vi "ROI to Default ROI Name.vi"(8 "Error In":errorcluster, 11 "ROI":T1) -> (0 "Error Out":errorcluster, 3 "ROI Type String":string)   [LabVIEW 2021, in "Image.lvlib"]
uses:
  Image.lvlib
panel:
  in  "Type":u32(ring)=1 items=["No Selection", "Point", "Line", "Rectangle", "Oval", "Polygon", "Free", "Annulus", "Unused2", "Unused3", "Broken Line", "Free Hand Line", "Rotated Rectangle"]
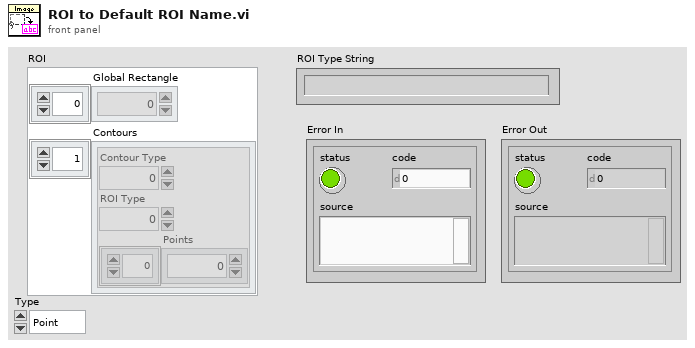
[diagram p1: front panel]
types:
  T1 = cluster{"Global Rectangle":i32[], "Contours":cluster{"Contour Type":u32, "ROI Type":u32, "Points":i32[]}[]}
  T2 = cluster{"Contour Type":u32, "ROI Type":u32, "Points":i32[]}[]
  T3 = cluster{"Contour Type":u32, "ROI Type":u32, "Points":i32[]}
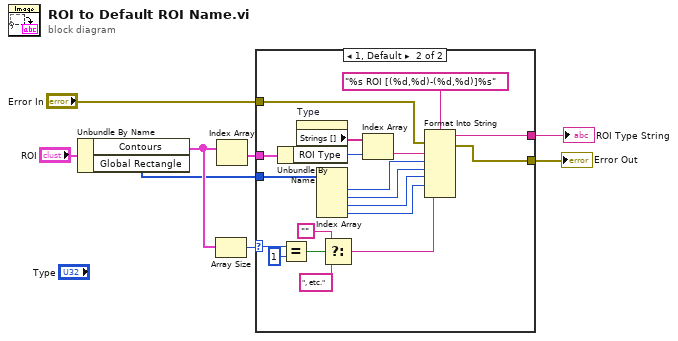
[diagram p0: block diagram]
diagram:
  n1 = Unbundle By Name("ROI") -> ("Contours"=w6:T2, "Global Rectangle"=w4:i32[])
  n2 = Array Size(array=w6) -> (size(s)=w5:i32)
  n3 = Index Array(array=w6) -> (element=w7:T3)  [unwired: 1 in]
  n4 = case shown="1, Default" w5 {
    selector: w5 -> [_ w23]
    tunnel: w7 -> [_ w24]
    tunnel: w4 -> [_ w17]
    tunnel: [_ w12] -> w3
    tunnel: "Error In" -> [w9 w11]
    tunnel: [w9 w10] -> w1
    frame 0 {
    }
    frame 1, Default {
      n5 = Unbundle By Name(w24) -> ("ROI Type"=w28:u32)
      n6 = Equal?(x=w23, y=1) -> (x = y?=w21:bool)
      n7 = property on="Type" class="Ring (strict)"() -> ("Strings []"=w27:string[])  [unwired: 2 in, 2 out]
      n8 = Index Array(array=w17) -> (element #1=w16:i32, element #2=w15:i32, element #3=w14:i32, element #4=w13:i32)  [unwired: 4 in]
      n9 = Select(t="", s=w21, f=", etc.") -> (s? t:f=w20:string)
      n10 = Index Array(array=w27, index=w28) -> (element=w26:string)
      n11 = Format Into String(format string="%s ROI [(%d,%d)-(%d,%d)]%s", error in=w11, w26, w16, w15, w14, w13, w20) -> (resulting string=w12:string, error out=w10:errorcluster)  [unwired: 1 in]
    }
  }
  "ROI Type String" <- w3
  "Error Out" <- w1
